vi "CRYFlatten Statistic.vi"(11 "Statistics":T1) -> (3 "Flatten Statistics String":string)   [LabVIEW 2013]
uses:
  Typedef Control/CRYStatistic cluster.ctl
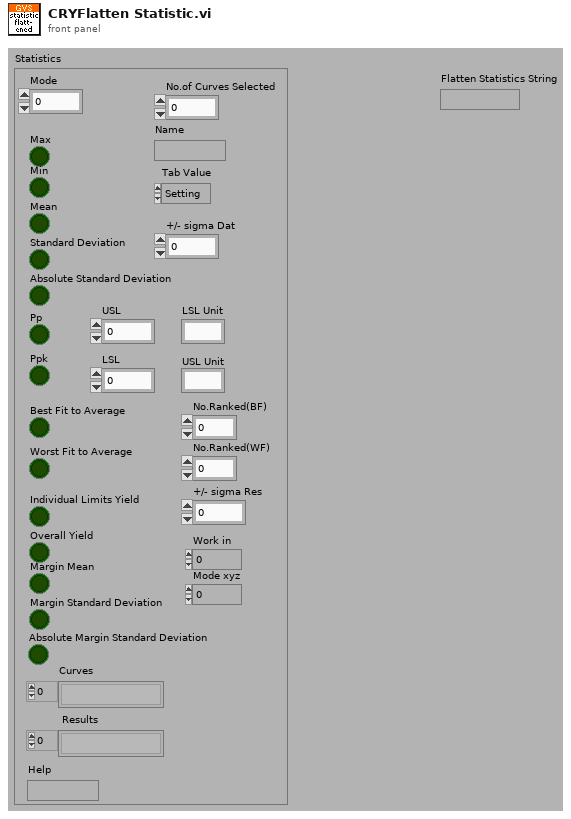
[diagram p1: front panel]
types:
  T1 = typedef "CRYStatistic cluster.ctl" = cluster{"Mode":u16, "No.Ranked(BF)":i32, "No.Ranked(WF)":i32, "Absolute Margin Standard Deviation":bool, "+/- sigma Res":i32, "Margin Standard Deviation":bool, "Margin Mean":bool, "Overall Yield":bool, "Individual Limits Yield":bool, "LSL Unit":string, "USL Unit\n":string, "LSL":dbl, "USL":dbl, "Worst Fit to Average":bool, "Best Fit to Average":bool, "Ppk":bool, "Pp":bool, "Absolute Standard Deviation":bool, "+/- sigma Dat":i32, "Standard Deviation ":bool, "Mean":bool, "Min ":bool, "Max ":bool, "No.of Curves Selected":i32, "Curves":string[], " Results":string[], "Name":string, "Help":string, "Tab Value":enum32{"Setting", "Help"}, "Work in":u16, "Mode xyz":u16}
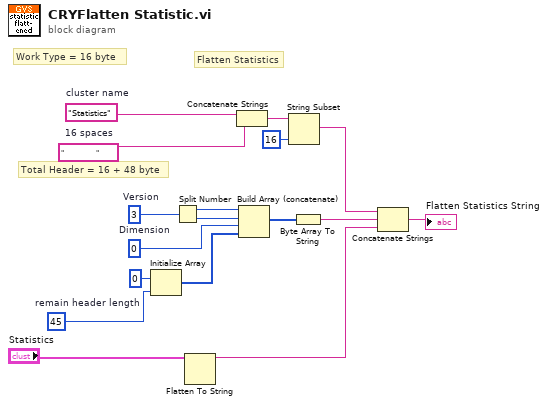
[diagram p0: block diagram]
diagram:
  w2 = "                "  # 16 spaces
  w3 = "Statistics"  # cluster name
  w8 = u16 3  # Version
  w11 = u8 0  # Dimension
  w7 = 45  # remain header length
  # "Flatten Statistics"
  # "Work Type = 16 byte"
  # "Total Header = 16 + 48 byte"
  n1 = Initialize Array(u8 0 ("element"), w7) -> (w13:u8[])
  n2 = Split Number(x=w8) -> (hi(x)=w9:u8, lo(x)=w10:u8)
  n3 = Flatten To String(anything="Statistics") -> (data string=w14:string)  [unwired: 1 in, 4 out]
  n4 = Concatenate Strings(w3, w2) -> (w4:string)
  n5 = Build Array (concatenate)(w9, w10, w11, w13) -> (w12:u8[])
  n6 = String Subset(string=w4, length (rest)=16 ("length (rest)")) -> (substring=w16:string)  [unwired: 1 out]
  n7 = Byte Array To String(unsigned byte array=w12) -> (string=w15:string)
  n8 = Concatenate Strings(w16, w15, w14) -> (→"Flatten Statistics String":string)
